vi "Log Loop.vi"(8 "error in (no error)":errorcluster) -> ()   [LabVIEW 2015]
uses:
  TypeDef/Log Actions.ctl
panel:
  in  "Target Directory":path=path "/home/lvuser/data"
  in  "Channel names":string[](array[string])
  in  "queue in":refnum<queue>
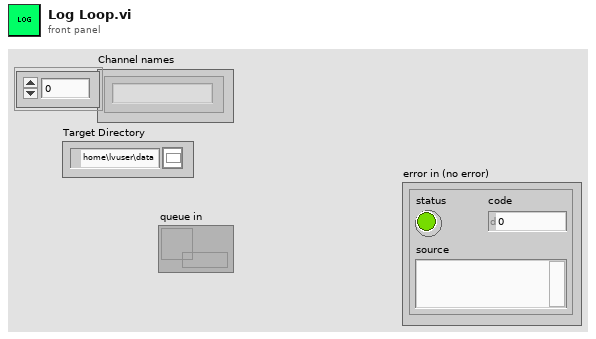
[diagram p1: front panel]
types:
  T1 = typedef "Log Actions.ctl" = enum16{"Remove oldest", "Open", "Log", "Check", "Close"}
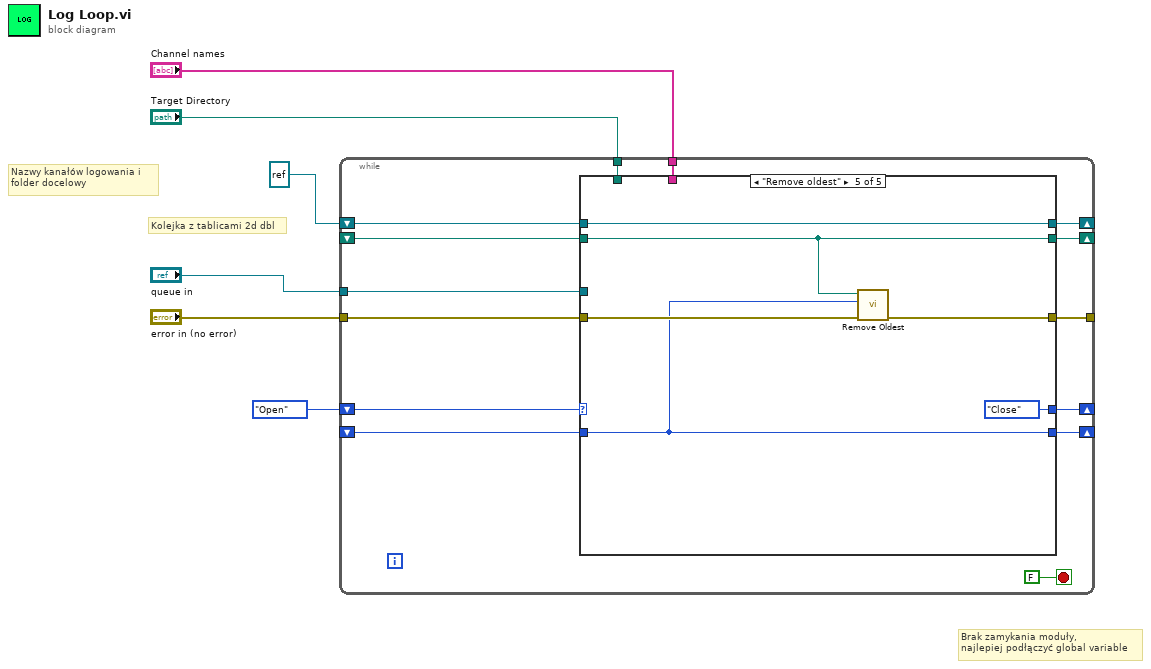
[diagram p0: block diagram]
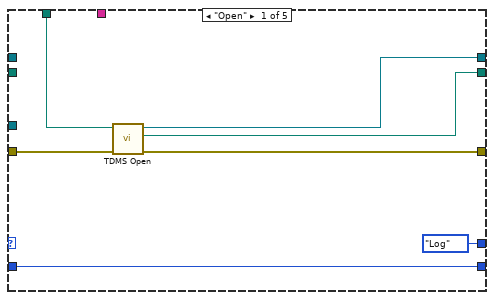
[diagram p2: hidden frame]
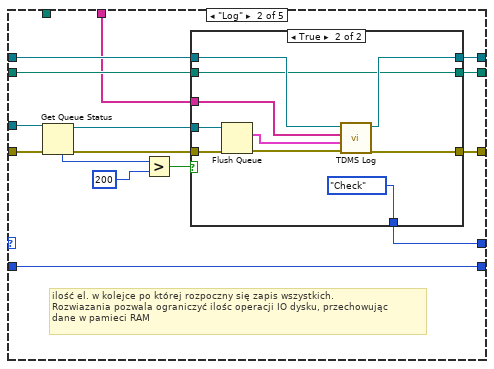
[diagram p3: hidden frame]
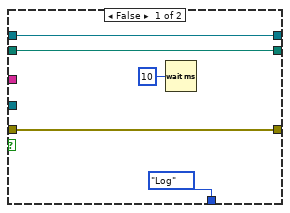
[diagram p4: hidden frame]
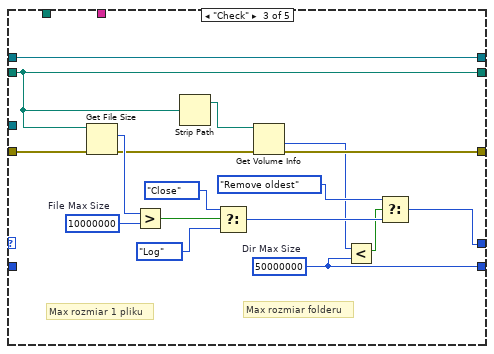
[diagram p5: hidden frame]
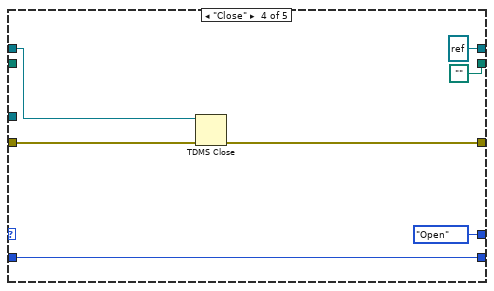
[diagram p6: hidden frame]
diagram:
  # "Nazwy kanałów logowania i\nfolder docelowy"
  # "Brak zamykania moduły,\nnajlepiej podłączyć global variable"
  # "Kolejka z tablicami 2d dbl"
  n1 = while {
    tunnel: "error in (no error)" -> [w17]
    tunnel: "queue in" -> [w18]
    shift-right: [w16] -> _
    shift-left: refnum<k34> refnum ("tdms file out") -> [w14]
    tunnel: [w15] -> _
    shift-right: [w13] -> _
    shift-left: Log_Actions."Open" -> [w20]
    shift-right: [w12] -> _
    shift-left: _ -> [w11]
    shift-right: [w10] -> _
    shift-left: _ -> [w9]
    tunnel: "Channel names" -> [w8]
    tunnel: "Target Directory" -> [w7]
    stop <- FALSE stop-if-true
    n2 = case shown="\"Remove oldest\"" w20 {
      tunnel: w18 -> [_ w41 _ _ _]
      tunnel: w17 -> [w27 w42 w74 w81 w87]
      tunnel: [w26 w33 w62 refnum<k34> refnum ("tdms file out") w83] -> w16
      tunnel: [w25 w34 w66 w80 w86] -> w15
      tunnel: w14 -> [_ w35 w62 w79 w83]
      tunnel: [Log_Actions."Log" w32 w61 Log_Actions."Open" Log_Actions."Close"] -> w13
      tunnel: [w23 w31 w63 path "" ("TDMS file path string") w82] -> w12
      tunnel: w11 -> [_ w30 w63 _ w82]
      tunnel: [w22 w29 w58 w75 w85] -> w10
      tunnel: w9 -> [w22 w29 _ w75 w85]
      tunnel: w8 -> [_ w28 _ _ _]
      tunnel: w7 -> [w21 _ _ _ _]
      frame "Open" {
        n3 = call "TDMS Open.vi"("error in (no error)"=w27, "File Path Control"=w21) -> ("error out"=w25:errorcluster, "TDMS file path string"=w23:path, "tdms file out"=w26:refnum<k34>)  [unwired: 7 in]
      }
      frame "Log" {
        # "ilość el. w kolejce po której rozpoczny się zapis wszystkich.\nRozwiazania pozwala ograniczyć ilośc operacji IO dysku, przechowując \ndane w pamieci RAM"
        n4 = Get Queue Status(queue=w41, error in (no error)=w42) -> (queue out=w36:refnum<queue>, error out=w37:errorcluster, # elements in queue=w40:i32)  [unwired: 1 in, 5 out]
        n5 = Greater?(x=w40, y=200) -> (0:w38:bool)
        n6 = case shown="True" w38 {
          tunnel: w37 -> [w47 w57]
          tunnel: w36 -> [_ w56]
          tunnel: w35 -> [w46 w54]
          tunnel: [w47 w55] -> w34
          tunnel: [w46 w53] -> w33
          tunnel: [Log_Actions."Log" Log_Actions."Check"] -> w32
          tunnel: w30 -> [w43 w51]
          tunnel: [w43 w51] -> w31
          tunnel: w28 -> [_ w49]
          frame False {
            n7 = Wait (ms)(milliseconds to wait=u32 10) -> ()  [unwired: 1 out]
          }
          frame True {
            n8 = Flush Queue(queue=w56, error in (no error)=w57) -> (remaining elements=w48:cluster{"Array":dbl[][]}[], error out=w50:errorcluster)  [unwired: 1 out]
            n9 = call "TDMS Log.vi"("error in"=w50, "Data"=w48, "Channel Names"=w49, "Refnum in"=w54) -> ("error out"=w55:errorcluster, "tdms file out"=w53:refnum<k34>)  [unwired: 6 in]
          }
        }
      }
      frame "Check" {
        w58 = i64 50000000  # Dir Max Size
        w72 = i64 10000000  # File Max Size
        # "Max rozmiar folderu"
        # "Max rozmiar 1 pliku"
        n10 = Get File Size(file=w63, error in=w74) -> (size (in bytes)=w73:i64, 0:w68:errorcluster)  [unwired: 1 out]
        n11 = Greater?(x=w73, y=w72) -> (0:w71:bool)
        n12 = Strip Path(path=w63) -> (stripped path=w67:path)  [unwired: 1 out]
        n13 = Select(t=Log_Actions."Close", s=w71, f=Log_Actions."Log") -> (s? t:f=w65:T1)
        n14 = Get Volume Info(8:w68, 11:w67) -> (0:w66:errorcluster, 1:w59:i64)  [unwired: 4 out]
        n15 = Less?(x=w59, y=w58) -> (x < y?=w60:bool)
        n16 = Select(t=Log_Actions."Remove oldest", s=w60, f=w65) -> (s? t:f=w61:T1)
      }
      frame "Close" {
        n17 = TDMS Close(8:w81, 11:w79) -> (0:w80:errorcluster)  [unwired: 1 out]
      }
      frame "Remove oldest" {
        n18 = call "Remove Oldest.vi"("error in (no error)"=w87, "Min volume free space"=w85, "TDMS file path string"=w82) -> ("Error Out"=w86:errorcluster)  [unwired: 8 in]
      }
    }
  }
